vi "Read Device Description XML.vi"(8 "error in (no error)":errorcluster, 11 "Device Description XML Path":path) -> (0 "error out":errorcluster, 1 "Device Data":variant, 2 "Config Pane Path":path, 3 "Device Name":string, 4 "Help Information":T1, 5 "Title Name":string, 6 "Weight":i32, 7 "Peripheral Name":string)   [LabVIEW 2021]
uses:
  <vilib>/xml/Load XML File.vi
  <vilib>/xml/Close Reference(Node).vi
  <vilib>/xml/NI_XML.lvlib
  <resource>/objmgr/DOMUserDefRef.rc
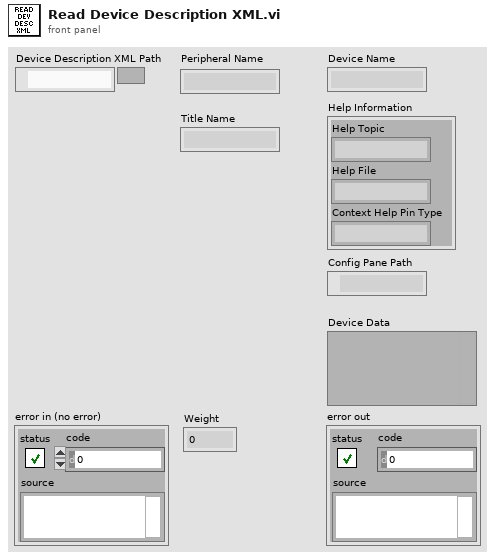
[diagram p1: front panel]
types:
  T1 = cluster{"Help Topic":string, "Help File":string, "Context Help Pin Type":string}
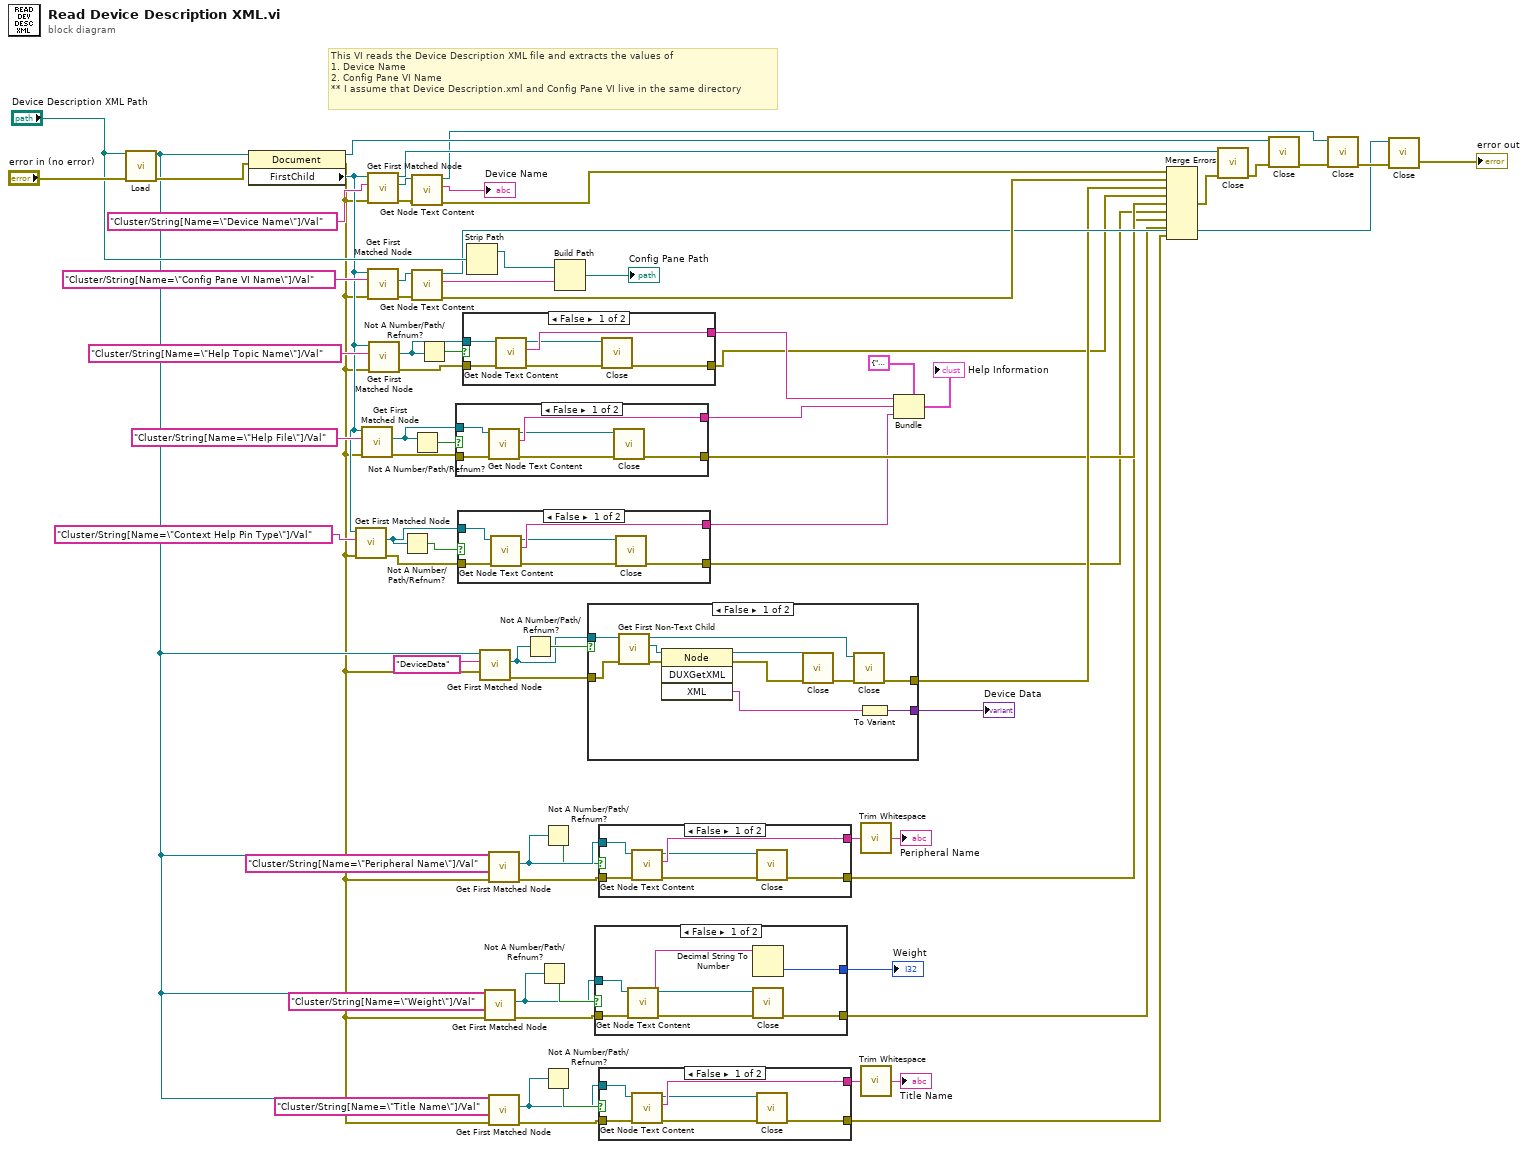
[diagram p0: block diagram]
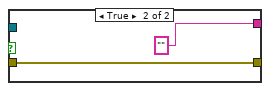
[diagram p2: hidden frame]
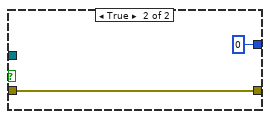
[diagram p3: hidden frame]
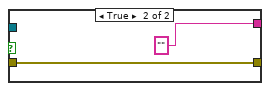
[diagram p4: hidden frame]
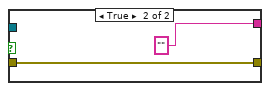
[diagram p5: hidden frame]
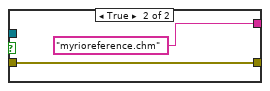
[diagram p6: hidden frame]
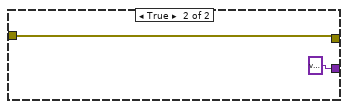
[diagram p7: hidden frame]
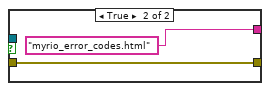
[diagram p8: hidden frame]
diagram:
  # "This VI reads the Device Description XML file and extracts the values of\n1. Device Name\n2. Config Pane VI Name\n** I assume that Device Description.xml and Config Pane VI live in the same directory"
  n1 = call-poly <vilib>:"Load.vi"("path to XML document"="Device Description XML Path", "error in (no error)"="error in (no error)") -> ("DOM document out"=w4:refnum<k20>, "error out"=w68:errorcluster)  [unwired: 11 in, 1 out]
  n2 = property class="Document"(reference=w4, error in=w68) -> (reference out=w63:refnum<k20>, error out=w3:errorcluster, "FirstChild"=w23:refnum<k20>)
  n3 = call <vilib>:"Get First Matched Node.vi"("error in (no error)"=w3, "XPath expression"="Cluster/String[Name=\"Context Help Pin Type\"]/Val", "node in"=w23) -> ("error out"=w25:errorcluster, "node result"=w28:refnum<k20>)  [unwired: 6 in, 1 out]
  n4 = call <vilib>:"Get First Matched Node.vi"("error in (no error)"=w3, "XPath expression"="Cluster/String[Name=\"Help File\"]/Val", "node in"=w23) -> ("error out"=w37:errorcluster, "node result"=w38:refnum<k20>)  [unwired: 6 in, 1 out]
  n5 = call <vilib>:"Get First Matched Node.vi"("error in (no error)"=w3, "XPath expression"="Cluster/String[Name=\"Device Name\"]/Val", "node in"=w23) -> ("error out"=w70:errorcluster, "node result"=w60:refnum<k20>, "node out"=w56:refnum<k20>)  [unwired: 6 in]
  n6 = call <vilib>:"Get First Matched Node.vi"("error in (no error)"=w3, "XPath expression"="Cluster/String[Name=\"Config Pane VI Name\"]/Val", "node in"=w23) -> ("error out"=w71:errorcluster, "node result"=w61:refnum<k20>)  [unwired: 6 in, 1 out]
  n7 = call <vilib>:"Get First Matched Node.vi"("error in (no error)"=w3, "XPath expression"="Cluster/String[Name=\"Help Topic Name\"]/Val", "node in"=w23) -> ("error out"=w46:errorcluster, "node result"=w45:refnum<k20>)  [unwired: 6 in, 1 out]
  n8 = Not A Number/Path/Refnum?(number/path/refnum=w28) -> (NaN/Path/Refnum?=w29:bool)
  n9 = call <vilib>:"Get Node Text Content.vi"("error in (no error)"=w70, "node in"=w60) -> ("error out"=w72:errorcluster, "node text"=→"Device Name":string, "node out"=w51:refnum<k20>)  [unwired: 7 in]
  n10 = call <vilib>:"Get Node Text Content.vi"("error in (no error)"=w71, "node in"=w61) -> ("error out"=w73:errorcluster, "node text"=w66:string, "node out"=w53:refnum<k20>)  [unwired: 7 in]
  n11 = Not A Number/Path/Refnum?(number/path/refnum=w38) -> (NaN/Path/Refnum?=w39:bool)
  n12 = Not A Number/Path/Refnum?(number/path/refnum=w45) -> (NaN/Path/Refnum?=w44:bool)
  n13 = case shown="False" w39 {
    tunnel: w37 -> [w79 w80]
    tunnel: [w78 "myrioreference.chm" ("node text")] -> w35
    tunnel: w38 -> [w77 _]
    tunnel: [w74 w80] -> w31
    frame False {
      n14 = call <vilib>:"Get Node Text Content.vi"("error in (no error)"=w79, "node in"=w77) -> ("error out"=w75:errorcluster, "node text"=w78:string, "node out"=w76:refnum<k20>)  [unwired: 7 in]
      n15 = call-poly <vilib>:"Close.vi"("error in (no error)"=w75, "node"=w76) -> ("error out"=w74:errorcluster)  [unwired: 7 in]
    }
    frame True {
    }
  }
  n16 = case shown="False" w29 {
    tunnel: [w87 "" ("node text")] -> w24
    tunnel: [w84 w88] -> w26
    tunnel: w28 -> [w83 _]
    tunnel: w25 -> [w82 w88]
    frame False {
      n17 = call <vilib>:"Get Node Text Content.vi"("error in (no error)"=w82, "node in"=w83) -> ("error out"=w85:errorcluster, "node text"=w87:string, "node out"=w86:refnum<k20>)  [unwired: 7 in]
      n18 = call-poly <vilib>:"Close.vi"("error in (no error)"=w85, "node"=w86) -> ("error out"=w84:errorcluster)  [unwired: 7 in]
    }
    frame True {
    }
  }
  n19 = case shown="False" w44 {
    tunnel: w46 -> [w95 w96]
    tunnel: [w94 "myrio_error_codes.html" ("node text")] -> w34
    tunnel: w45 -> [w93 _]
    tunnel: [w90 w96] -> w32
    frame False {
      n20 = call <vilib>:"Get Node Text Content.vi"("error in (no error)"=w95, "node in"=w93) -> ("error out"=w91:errorcluster, "node text"=w94:string, "node out"=w92:refnum<k20>)  [unwired: 7 in]
      n21 = call-poly <vilib>:"Close.vi"("error in (no error)"=w91, "node"=w92) -> ("error out"=w90:errorcluster)  [unwired: 7 in]
    }
    frame True {
    }
  }
  n22 = Strip Path(path="Device Description XML Path") -> (stripped path=w64:path)  [unwired: 1 out]
  n23 = call <vilib>:"Get First Matched Node.vi"("error in (no error)"=w3, "XPath expression"="DeviceData", "node in"=w4) -> ("error out"=w42:errorcluster, "node result"=w40:refnum<k20>)  [unwired: 6 in, 1 out]
  n24 = call <vilib>:"Get First Matched Node.vi"("error in (no error)"=w3, "XPath expression"="Cluster/String[Name=\"Weight\"]/Val", "node in"=w4) -> ("error out"=w12:errorcluster, "node result"=w14:refnum<k20>)  [unwired: 6 in, 1 out]
  n25 = call <vilib>:"Get First Matched Node.vi"("error in (no error)"=w3, "XPath expression"="Cluster/String[Name=\"Peripheral Name\"]/Val", "node in"=w4) -> ("error out"=w22:errorcluster, "node result"=w17:refnum<k20>)  [unwired: 6 in, 1 out]
  n26 = call <vilib>:"Get First Matched Node.vi"("error in (no error)"=w3, "XPath expression"="Cluster/String[Name=\"Title Name\"]/Val", "node in"=w4) -> ("error out"=w5:errorcluster, "node result"=w8:refnum<k20>)  [unwired: 6 in, 1 out]
  n27 = Not A Number/Path/Refnum?(number/path/refnum=w40) -> (NaN/Path/Refnum?=w41:bool)
  n28 = Not A Number/Path/Refnum?(number/path/refnum=w14) -> (NaN/Path/Refnum?=w15:bool)
  n29 = Not A Number/Path/Refnum?(number/path/refnum=w17) -> (NaN/Path/Refnum?=w16:bool)
  n30 = Not A Number/Path/Refnum?(number/path/refnum=w8) -> (NaN/Path/Refnum?=w9:bool)
  n31 = Build Path(base path=w64, name or relative path=w66) -> (appended path=→"Config Pane Path":path)
  n32 = case shown="False" w41 {
    tunnel: w42 -> [w104 w110]
    tunnel: [w108 variant ("Variant")] -> w49
    tunnel: [w99 w110] -> w48
    tunnel: w40 -> [w107 _]
    frame False {
      n33 = call <vilib>:"Get First Non-Text Child.vi"("error in (no error)"=w104, "node in"=w107) -> ("error out"=w103:errorcluster, "child node"=w106:refnum<k20>, "node out"=w98:refnum<k20>)  [unwired: 6 in, 1 out]
      n34 = invoke class="Node" method="DUXGetXML"(reference=w106, error in=w103) -> (reference out=w101:refnum<k20>, error out=w102:errorcluster, "XML"=w105:string)  [unwired: 2 in, 1 out]
      n35 = call-poly <vilib>:"Close.vi"("error in (no error)"=w102, "node"=w101) -> ("error out"=w100:errorcluster)  [unwired: 7 in]
      n36 = call-poly <vilib>:"Close.vi"("error in (no error)"=w100, "node"=w98) -> ("error out"=w99:errorcluster)  [unwired: 7 in]
      n37 = To Variant(anything=w105) -> (Variant=w108:variant)
    }
    frame True {
    }
  }
  "Device Data" <- w49
  n38 = case shown="False" w15 {
    tunnel: [w115 w119] -> w10
    tunnel: w14 -> [w114 _]
    tunnel: w12 -> [w113 w119]
    tunnel: [w112 0] -> w11
    frame False {
      n39 = call <vilib>:"Get Node Text Content.vi"("error in (no error)"=w113, "node in"=w114) -> ("error out"=w116:errorcluster, "node text"=w111:string, "node out"=w117:refnum<k20>)  [unwired: 7 in]
      n40 = Decimal String To Number(string=w111) -> (number=w112:i32)  [unwired: 2 in, 1 out]
      n41 = call-poly <vilib>:"Close.vi"("error in (no error)"=w116, "node"=w117) -> ("error out"=w115:errorcluster)  [unwired: 7 in]
    }
    frame True {
    }
  }
  "Weight" <- w11
  n42 = case shown="False" w16 {
    tunnel: [w125 "" ("node text")] -> w21
    tunnel: [w122 w126] -> w18
    tunnel: w17 -> [w121 _]
    tunnel: w22 -> [w120 w126]
    frame False {
      n43 = call <vilib>:"Get Node Text Content.vi"("error in (no error)"=w120, "node in"=w121) -> ("error out"=w123:errorcluster, "node text"=w125:string, "node out"=w124:refnum<k20>)  [unwired: 7 in]
      n44 = call-poly <vilib>:"Close.vi"("error in (no error)"=w123, "node"=w124) -> ("error out"=w122:errorcluster)  [unwired: 7 in]
    }
    frame True {
    }
  }
  n45 = case shown="False" w9 {
    tunnel: [w133 "" ("node text")] -> w6
    tunnel: [w130 w134] -> w1
    tunnel: w8 -> [w129 _]
    tunnel: w5 -> [w128 w134]
    frame False {
      n46 = call <vilib>:"Get Node Text Content.vi"("error in (no error)"=w128, "node in"=w129) -> ("error out"=w131:errorcluster, "node text"=w133:string, "node out"=w132:refnum<k20>)  [unwired: 7 in]
      n47 = call-poly <vilib>:"Close.vi"("error in (no error)"=w131, "node"=w132) -> ("error out"=w130:errorcluster)  [unwired: 7 in]
    }
    frame True {
    }
  }
  n48 = call <vilib>:"Trim Whitespace.vi"("string"=w21) -> ("trimmed string"=→"Peripheral Name":string)  [unwired: 1 in]
  n49 = call <vilib>:"Trim Whitespace.vi"("string"=w6) -> ("trimmed string"=→"Title Name":string)  [unwired: 1 in]
  n50 = Bundle(cluster=T1 {"Help Topic"="", "Help File"="", "Context Help Pin Type"=""}, "Help Topic"=w34, "Help File"=w35, "Context Help Pin Type"=w24) -> (→"Help Information":T1)
  n51 = Merge Errors(w72, w73, w48, w32, w31, w26, w18, w10, w1) -> (w58:errorcluster)
  n52 = call-poly <vilib>:"Close.vi"("error in (no error)"=w58, "node"=w56) -> ("error out"=w57:errorcluster)  [unwired: 7 in]
  n53 = call-poly <vilib>:"Close.vi"("error in (no error)"=w57, "node"=w63) -> ("error out"=w55:errorcluster)  [unwired: 7 in]
  n54 = call-poly <vilib>:"Close.vi"("error in (no error)"=w55, "node"=w51) -> ("error out"=w54:errorcluster)  [unwired: 7 in]
  n55 = call-poly <vilib>:"Close.vi"("error in (no error)"=w54, "node"=w53) -> ("error out"=→"error out":errorcluster)  [unwired: 7 in]
